vi "points2code.vi"(11 "Array in":T1[](array[typedef])) -> (3 "Array out":string[](array[string]))   [LabVIEW 2021]
uses:
  <vilib>/Utility/miscctls.llb/LVPoint32TypeDef.ctl
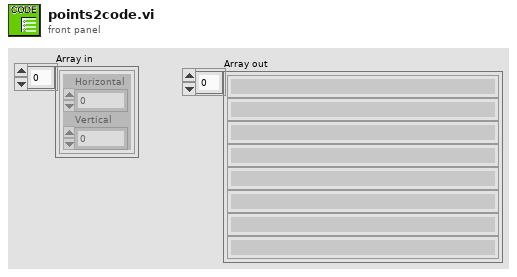
[diagram p1: front panel]
types:
  T1 = typedef "LVPoint32TypeDef.ctl" = cluster{"Horizontal":i32, "Vertical":i32}
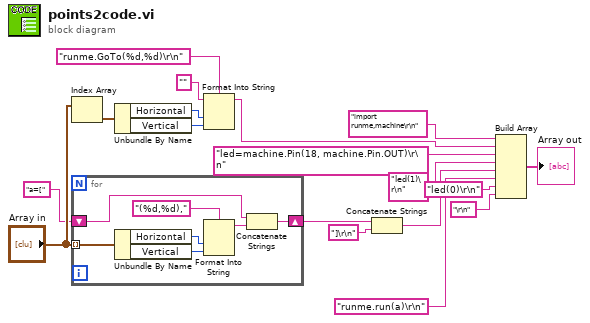
[diagram p0: block diagram]
diagram:
  n1 = Index Array(array="Array in") -> (element=w12:T1)  [unwired: 1 in]
  n2 = for {
    tunnel: "Array in" -> [w25] mode=indexing
    shift-right: [w19] -> w17
    shift-left: "a=[" -> [w20]
    n3 = Unbundle By Name(w25) -> ("Horizontal"=w23:i32, "Vertical"=w22:i32)
    n4 = Format Into String(format string="(%d,%d),", w23, w22) -> (resulting string=w21:string)  [unwired: 2 in, 1 out]
    n5 = Concatenate Strings(w20, w21) -> (w19:string)
  }
  n6 = Unbundle By Name(w12) -> ("Horizontal"=w14:i32, "Vertical"=w15:i32)
  n7 = Format Into String(format string="runme.GoTo(%d,%d)\r\n", initial string="", w14, w15) -> (resulting string=w3:string)  [unwired: 1 in, 1 out]
  n8 = Concatenate Strings(w17, "]\r\n" ("string")) -> (w18:string)
  n9 = Build Array("import runme,machine\r\n", w3, "led=machine.Pin(18, machine.Pin.OUT)\r\n" ("element"), "led(1)\r\n" ("element"), w18, "runme.run(a)\r\n", "led(0)\r\n" ("element"), "\r\n" ("element")) -> (→"Array out":string[])
